vi "AirmarQuickTestLoop.vi"() -> ()   [LabVIEW 2012]
uses:
  2-Think/2 Typedefs/UTM Location.ctl
  2-Think/2 Globals/2 Global.vi
panel:
  out "Location":cluster{dbl[], dbl[]}(graph)
  out "Absolute Wind Direction":dbl(graph)
  out "Robot UTM Location":T1 {"North" format="%#_10f"; "East" format="%#_8f"}
  in  "VISA Refnum in":refnum<visa-resource-name>="COM1"
  in  "stop":bool
  # "Set this before running!"
  # "Don't run at same time as actual robot code."
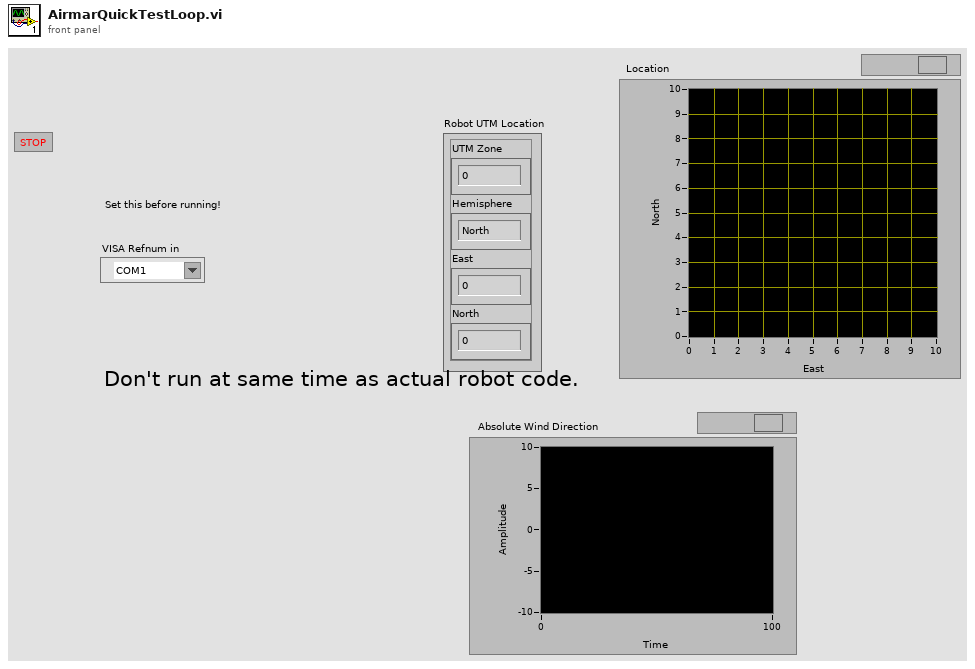
[diagram p1: front panel]
types:
  T1 = typedef "UTM Location.ctl" = cluster{"UTM Zone":dbl, "Hemisphere":enum16{"North", "South"}, "East":dbl, "North":dbl}
  T2 = typedef "absolute wind direction.ctl" = dbl
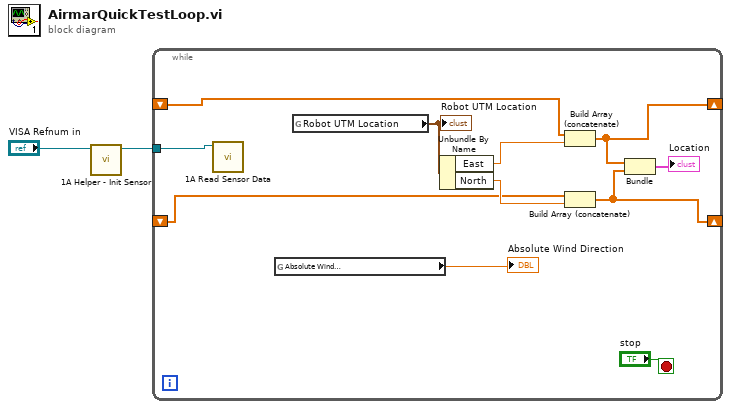
[diagram p0: block diagram]
diagram:
  n1 = call "1A Helper - Init Sensor.vi"("VISA Refnum in"="VISA Refnum in") -> ("VISA Refnum out"=w1:refnum<visa-resource-name>)  [unwired: 8 in, 2 out]
  n2 = while {
    tunnel: w1 -> [w12]
    shift-right: [w5] -> _
    shift-left: _ -> [w8]
    shift-right: [w4] -> _
    shift-left: _ -> [w6]
    stop <- "stop" stop-if-true
    n3 = call "1A Read Sensor Data.vi"("VISA resource name (in)"=w12) -> ()  [unwired: 9 in, 2 out]
    n4 = global read "2 Global.vi" "Absolute Wind\nDirection (º)"() -> (→"Absolute Wind Direction":T2)
    n5 = global read "2 Global.vi" "Robot UTM Location"() -> (w10:T1)
    "Robot UTM Location" <- w10
    n6 = Unbundle By Name(w10) -> ("East"=w9:dbl, "North"=w7:dbl)
    n7 = Build Array (concatenate)(w8, w9) -> (w5:dbl[])
    n8 = Build Array (concatenate)(w6, w7) -> (w4:dbl[])
    n9 = Bundle(w5, w4) -> (→"Location":cluster{dbl[], dbl[]})  [unwired: 1 in]
  }
